vi "Write-Data.vi"(8 "error in (no error)":errorcluster, 10 "Data":dbl[](array[numeric]), 11 "Type-K-Thermocouple in":refnum<class "Pressure-Transducer.lvclass">) -> (0 "error out":errorcluster, 3 "Type-K-Thermocouple out":refnum<class "Pressure-Transducer.lvclass">)   [LabVIEW 2021, in "Pressure-Transducer.lvclass"]
uses:
  Pressure-Transducer.lvclass
  Modbus-Instr_class/Modbus-Instr.lvclass
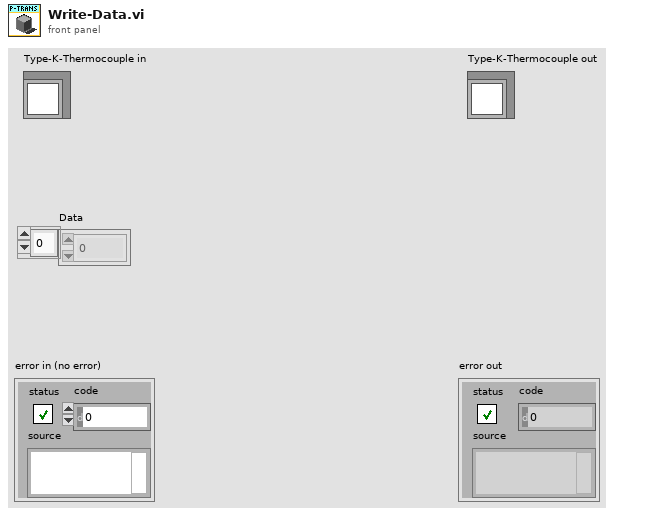
[diagram p1: front panel]
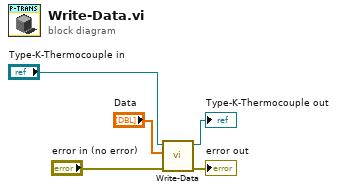
[diagram p0: block diagram]
diagram:
  n1 = call-parent "Write-Data.vi"("error in (no error)"="error in (no error)", "Data"="Data", "Modbus-Instr in"="Type-K-Thermocouple in") -> ("error out"=→"error out":errorcluster, "Modbus-Instr out"=→"Type-K-Thermocouple out":refnum<class "Pressure-Transducer.lvclass">)  [unwired: 7 in]
